vi "TestExec.Variant to 1D Str Args.vi"(10 "Default Args":string[](array[string]), 11 "Variant":variant) -> (2 "Empty":bool, 3 "Args":string[](array[string]))   [LabVIEW 2019]
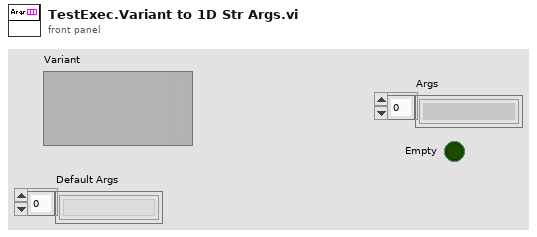
[diagram p1: front panel]
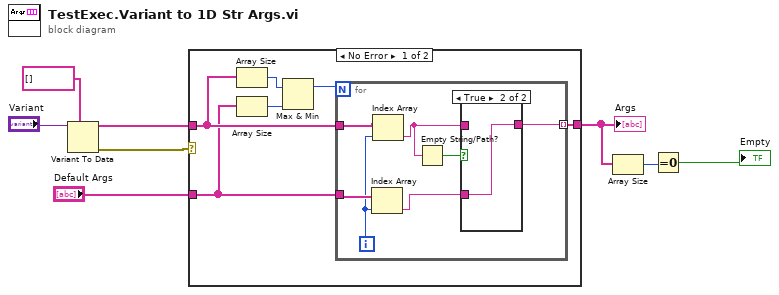
[diagram p0: block diagram]
diagram:
  n1 = Variant To Data(type=string[] [] ("Args"), Variant="Variant") -> (data=w2:string[], error out=w6:errorcluster)  [unwired: 1 in]
  n2 = case shown="No Error" w6 {
    tunnel: w2 -> [w10 _]
    tunnel: [w14 w24] -> w5
    tunnel: "Default Args" -> [w9 w24]
    frame No Error {
      n3 = Array Size(array=w10) -> (size(s)=w12:i32)
      n4 = Array Size(array=w9) -> (size(s)=w13:i32)
      n5 = Max & Min(x=w12, y=w13) -> (max(x,y)=w11:i32)  [unwired: 1 out]
      n6 = for {
        N: w11 -> [_]
        tunnel: w10 -> [w17]
        tunnel: w9 -> [w18]
        tunnel: [w20] -> w14 mode=indexing
        i -> [w15]
        n7 = Index Array(array=w18, index=w15) -> (element=w19:string)
        n8 = Index Array(array=w17, index=w15) -> (element=w16:string)
        n9 = Empty String/Path?(string/path=w16) -> (empty?=w21:bool)
        n10 = case shown="True" w21 {
          tunnel: w16 -> [w22 _]
          tunnel: [w22 w23] -> w20
          tunnel: w19 -> [_ w23]
          frame False {
          }
          frame True {
          }
        }
      }
    }
    frame Error {
    }
  }
  "Args" <- w5
  n11 = Array Size(array=w5) -> (size(s)=w4:i32)
  n12 = Equal To 0?(x=w4) -> (x = 0?=→"Empty":bool)
